vi "load-robot-vr.vi"(8 "错误输入":errorcluster) -> (0 "错误输出":errorcluster)   [LabVIEW 2013]
uses:
  <vilib>/picture/3D Picture Control/NI_3D Picture Control.lvlib
panel:
  out "ZuoHouRef":T1
  in  "ZuoHou":T1
  out "YouHouRef":T2
  in  "YouHou":T2
  out "YouQianRef":T3
  in  "YouQian":T3
  out "ZuoQianRef":T4
  in  "ZuoQian":T4
  out "BodyRef":refnum<vi>
  out "RobotRef":refnum<vi>
  out "Display":refnum<vi>(3d-picture)
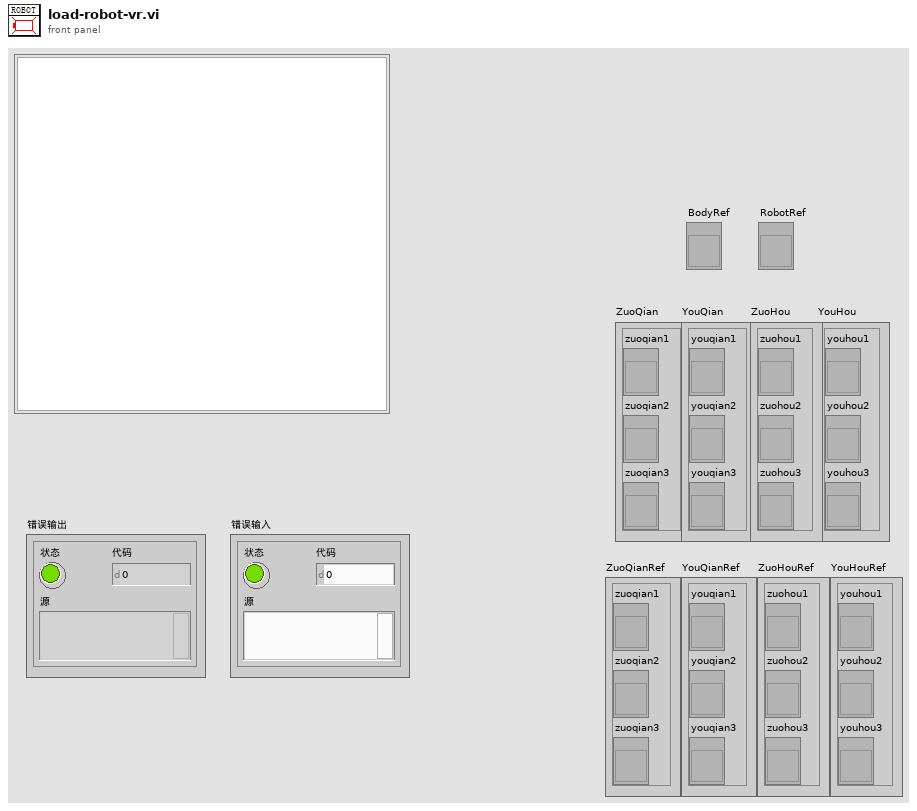
[diagram p1: front panel]
types:
  T1 = cluster{"zuohou1":refnum<vi>, "zuohou2":refnum<vi>, "zuohou3":refnum<vi>}
  T2 = cluster{"youhou1":refnum<vi>, "youhou2":refnum<vi>, "youhou3":refnum<vi>}
  T3 = cluster{"youqian1":refnum<vi>, "youqian2":refnum<vi>, "youqian3":refnum<vi>}
  T4 = cluster{"zuoqian1":refnum<vi>, "zuoqian2":refnum<vi>, "zuoqian3":refnum<vi>}
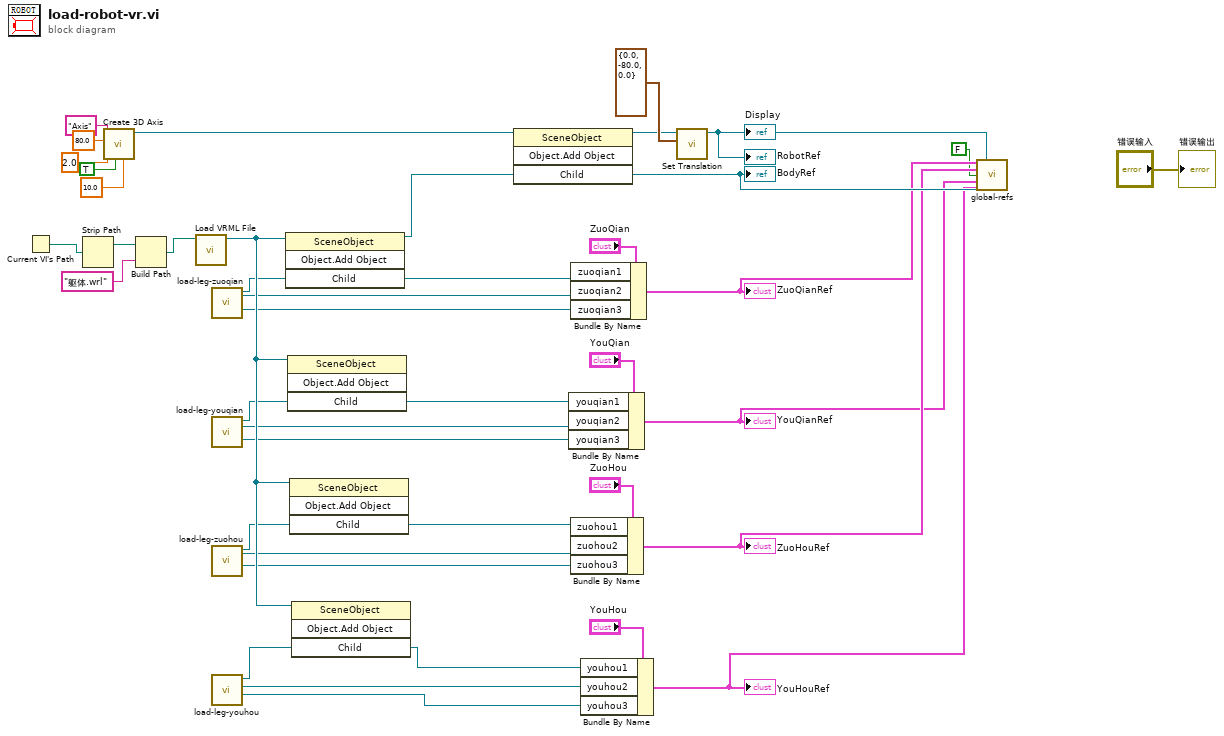
[diagram p0: block diagram]
diagram:
  n1 = Current VI's Path() -> (path=w38:path)
  n2 = Strip Path(path=w38) -> (stripped path=w35:path)  [unwired: 1 out]
  n3 = call <vilib>:"Create 3D Axis.vi"("Character Size"=sgl 10.0, "Axis label?"=TRUE, "Radius"=sgl 2.0, "Length"=sgl 80.0, "Name"="Axis") -> ("New Object Refnum"=w34:refnum<vi>)  [unwired: 5 in, 1 out]
  n4 = Build Path(base path=w35, name or relative path="躯体.wrl" ("名称或相对路径")) -> (appended path=w37:path)
  n5 = call <vilib>:"Load VRML File.vi"("Path"=w37) -> ("Scene:Read Scene File"=w33:refnum<vi>)  [unwired: 9 in, 1 out]
  n6 = call "load-leg-zuoqian.vi"() -> ("zuoqian3"=w24:refnum<vi>, "zuoqian2"=w25:refnum<vi>, "zuoqian1"=w32:refnum<vi>)  [unwired: 8 in, 1 out]
  n7 = call "load-leg-youqian.vi"() -> ("youqian3"=w20:refnum<vi>, "youqian2"=w21:refnum<vi>, "youqian1"=w31:refnum<vi>)  [unwired: 8 in, 1 out]
  n8 = call "load-leg-zuohou.vi"() -> ("zuohou3"=w12:refnum<vi>, "zuohou2"=w13:refnum<vi>, "zuohou1"=w30:refnum<vi>)  [unwired: 8 in, 1 out]
  n9 = call "load-leg-youhou.vi"() -> ("youhou3"=w16:refnum<vi>, "youhou2"=w17:refnum<vi>, "youhou1"=w29:refnum<vi>)  [unwired: 8 in, 1 out]
  n10 = invoke class="SceneObject" method="Object.Add Object"(reference=w33, "Child"=w32) -> (reference out=w28:refnum<vi>, "Child"=w26:refnum<vi>)  [unwired: 2 in, 2 out]
  n11 = invoke class="SceneObject" method="Object.Add Object"(reference=w33, "Child"=w31) -> ("Child"=w22:refnum<vi>)  [unwired: 2 in, 3 out]
  n12 = invoke class="SceneObject" method="Object.Add Object"(reference=w33, "Child"=w30) -> ("Child"=w14:refnum<vi>)  [unwired: 2 in, 3 out]
  n13 = invoke class="SceneObject" method="Object.Add Object"(reference=w33, "Child"=w29) -> ("Child"=w18:refnum<vi>)  [unwired: 2 in, 3 out]
  n14 = invoke class="SceneObject" method="Object.Add Object"(reference=w34, "Child"=w28) -> (reference out=w2:refnum<vi>, "Child"=w11:refnum<vi>)  [unwired: 2 in, 2 out]
  "BodyRef" <- w11
  n15 = Bundle By Name(cluster="YouQian", "youqian1"=w22, "youqian2"=w21, "youqian3"=w20) -> (w8:T3)
  "YouQianRef" <- w8
  n16 = Bundle By Name(cluster="ZuoQian", "zuoqian1"=w26, "zuoqian2"=w25, "zuoqian3"=w24) -> (w10:T4)
  "ZuoQianRef" <- w10
  n17 = Bundle By Name(cluster="ZuoHou", "zuohou1"=w14, "zuohou2"=w13, "zuohou3"=w12) -> (w9:T1)
  "ZuoHouRef" <- w9
  n18 = Bundle By Name(cluster="YouHou", "youhou1"=w18, "youhou2"=w17, "youhou3"=w16) -> (w7:T2)
  "YouHouRef" <- w7
  n19 = call <vilib>:"Set Translation.vi"("Translation"=cluster{"X":sgl, "Y":sgl, "Z":sgl} {"X"=0.0, "Y"=-80.0, "Z"=0.0}, "Scene Object"=w2) -> ("Translated Object"=w1:refnum<vi>)  [unwired: 8 in, 1 out]
  "Display" <- w1
  "RobotRef" <- w1
  n20 = call "global-refs.vi"("ZuoQian"=w10, "Robot"=w1, "ZuoHou"=w9, "Read?"=FALSE, "YouQian"=w8, "YouHou"=w7, "Body"=w11) -> ()  [unwired: 3 in, 6 out]
  "错误输出" <- "错误输入"
